vi "VCI_GetReference.vi"(7 "RegistID":u8, 8 "error in (no error)":errorcluster caption="错误输入（无错误）", 9 "CANIndex":u32, 10 "DevIndex":u32, 11 "DevType":T1=2 items=["USB-CAN"=2, "USB-CAN2"=3]) -> (0 "error out":errorcluster caption="错误输出", 2 "pData":u8[](array[numeric]), 3 "Return Val":T2=1 items=["OK"=1, "ERROR1"=0, "ERROR2"=-1])   [LabVIEW 2018, in "ControlCan.lvlib"]
uses:
  ControlCan.lvlib
  Return Val.ctl
  DevType.ctl
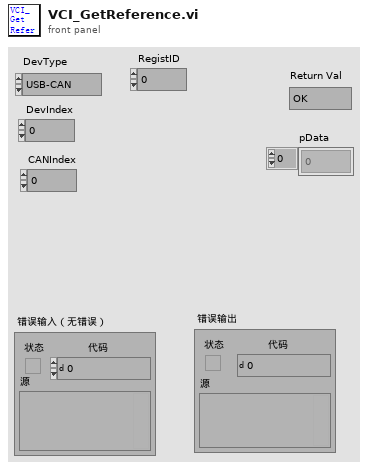
[diagram p1: front panel]
types:
  T1 = typedef "ControlCAN.lvlib/DevType.ctl" = u32
  T2 = typedef "ControlCAN.lvlib/Return Val.ctl" = i32
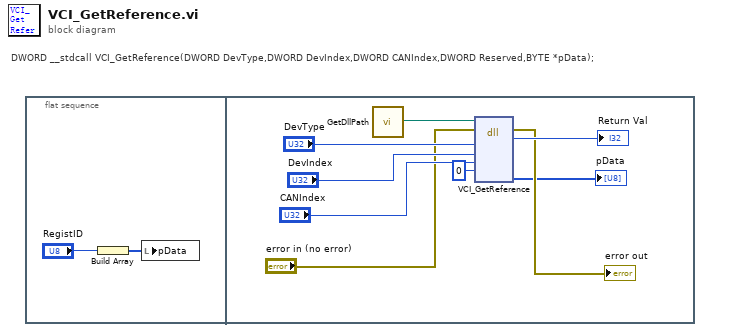
[diagram p0: block diagram]
diagram:
  # "DWORD __stdcall VCI_GetReference(DWORD DevType,DWORD DevIndex,DWORD CANIndex,DWORD Reserved,BYTE *pData);"
  n1 = flat-sequence {
    frame #0 {
      n2 = Build Array("RegistID") -> (w2:u8[])
      n3 = local write "pData"(w2) -> ()
    }
    frame #1 {
      n4 = call "GetDllPath.vi"() -> ("DllPath"=w3:path)  [unwired: 1 in]
      n5 = dll-call lib="?" fn="VCI_GetReference"(path in=w3, error in="error in (no error)", "DevType"="DevType", "DevIndex"="DevIndex", "CANIndex"="CANIndex", "Reserved"=u32 0) -> (error out=→"error out":errorcluster, "ReturnVal"=→"Return Val":i32, "pData"=→"pData":u8[])  [unwired: 6 in, 1 out]
    }
  }
